vi "Write nextInChain.vi"(8 "error in (no error)":errorcluster, 10 "Chain.lvclass":refnum<class "Chain.lvclass">, 11 "Chain in":refnum<class "Chain.lvclass">) -> (0 "error out":errorcluster, 3 "Chain out":refnum<class "Chain.lvclass">)   [LabVIEW 2017, in "Chain.lvclass"]
uses:
  Chain.lvclass
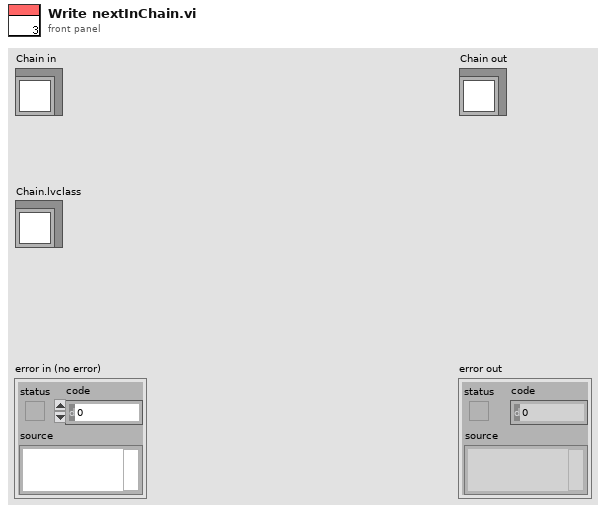
[diagram p1: front panel]
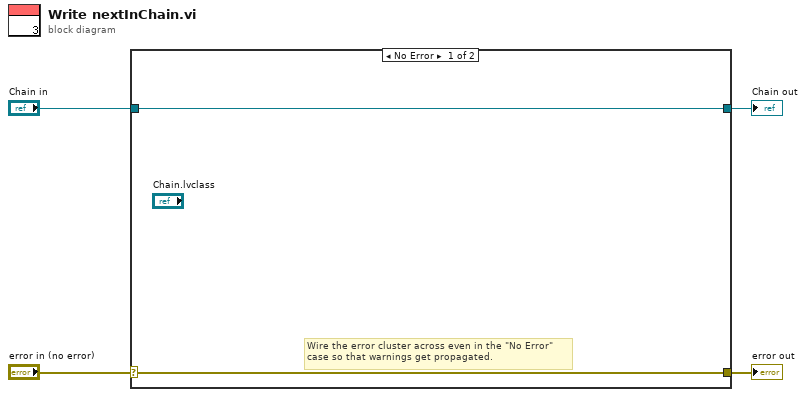
[diagram p0: block diagram]
diagram:
  n1 = case shown="No Error" "error in (no error)" {
    selector: "error in (no error)" -> [w5 w8]
    tunnel: [w5 w8] -> w3
    tunnel: [w6 w7] -> w1
    tunnel: "Chain in" -> [w6 w7]
    frame No Error {
      # "Wire the error cluster across even in the \"No Error\"\ncase so that warnings get propagated."
    }
    frame Error {
    }
  }
  "error out" <- w3
  "Chain out" <- w1
